vi "Pre Launch Init.vi"(11 "ParentActor in":refnum<class "ParentActor.lvclass">) -> (0 "error out":errorcluster, 3 "ParentActor out":refnum<class "ParentActor.lvclass">)   [LabVIEW 2020, in "ParentActor.lvclass"]
doc: "(<B>Filename</B>: Actor Framework.lvlib:Actor.lvclass:Pre Launch Init.vi)\n\nDefines behavior that occurs after the Launch Nested Actor method is invoked but before the actor's Actor Core method begins running.\n\nBy default, this method does nothing. A descendant class may override it to define behavior."
uses:
  ParentActor/ParentActor.lvclass
  ParentActor/ParentActor.lvclass/ParentActor.ctl
  <vilib>/ActorFramework/Actor/Actor.lvclass
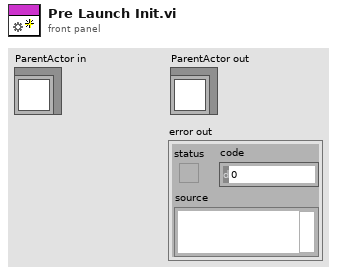
[diagram p1: front panel]
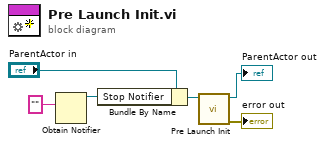
[diagram p0: block diagram]
diagram:
  n1 = Obtain Notifier(notification data type="" ("name (unnamed)")) -> (notifier out=w3:refnum<notifier>)  [unwired: 3 in, 2 out]
  n2 = Bundle By Name(cluster="ParentActor in", "Stop Notifier"=w3) -> (w2:refnum<class "ParentActor.lvclass">)
  n3 = call-parent "Pre Launch Init.vi"("Actor in"=w2) -> ("error out"=→"error out":errorcluster, "Actor out"=→"ParentActor out":refnum<class "ParentActor.lvclass">)  [unwired: 9 in]
